vi "rotate_nicks_bot.vi"(8 "degrees to  rotate":dbl, 9 "right(T)/left(F)":bool, 10 "power":u16=75, 11 "NXT 2":T1={"Hardware"="NXT", "Flattened String"=""}) -> (3 "NXT":T1={"Hardware"="NXT", "Flattened String"=""})   [LabVIEW 2012]
uses:
  <vilib>/NXT/Subs/LVHSConnector.ctl
  <vilib>/NXT/Subs/MotorOutput.ctl
  <vilib>/NXT/Dual Mode Library/Motors/MotorBrake.vi
  <vilib>/NXT/Dual Mode Library/Display/drawText.vi
  <vilib>/NXT/Dual Mode Library/Waits/Wait_Num.vi
  <vilib>/NXT/Dual Mode Library/Motors/MotorOn.vi
  <vilib>/NXT/Dual Mode Library/Motors/MotorReverse.vi
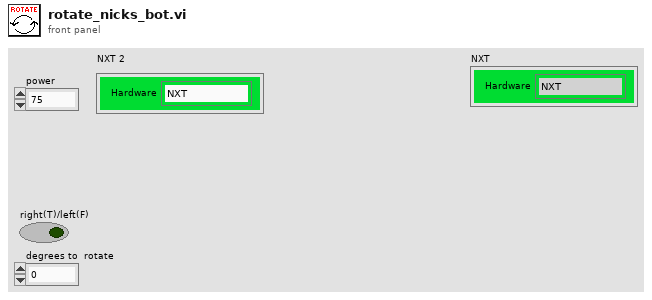
[diagram p1: front panel]
types:
  T1 = typedef "LVHSConnector.ctl" = cluster{"Hardware":string, "Flattened String":string}
  T2 = typedef "MotorOutput.ctl" = u8
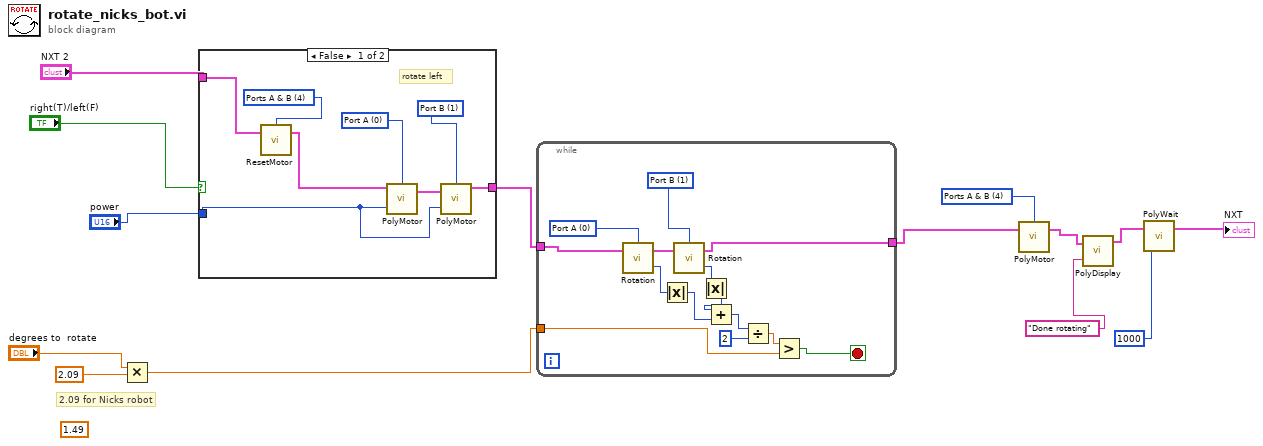
[diagram p0: block diagram]
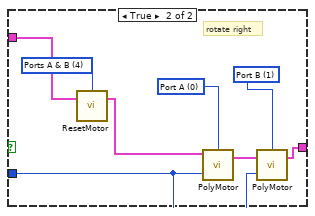
[diagram p2: hidden frame]
diagram:
  (unwired) 1.49 ("Max Value")
  w1 = T2 4 items=["Port A"=0, "Port B"=1, "Port C"=2, "Ports A & B"=4, "Ports A & C"=5, "Ports B & C"=6, "All Ports"=3] ("Port (All Ports)")
  # "2.09 for Nicks robot"
  n1 = Multiply(x="degrees to  rotate", y=2.09 ("Max Value")) -> (x*y=w10:dbl)
  n2 = case shown="False" "right(T)/left(F)" {
    tunnel: "power" -> [w15 w23]
    tunnel: "NXT 2" -> [w19 w25]
    tunnel: [w17 w24] -> w8
    frame False {
      w16 = T2 4 items=["Port A"=0, "Port B"=1, "Port C"=2, "Ports A & B"=4, "Ports A & C"=5, "Ports B & C"=6, "All Ports"=3] ("Port (All Ports)")
      w22 = T2 1 items=["Port A"=0, "Port B"=1, "Port C"=2, "Ports A & B"=4, "Ports A & C"=5, "Ports B & C"=6, "as"=3] ("Output Port (All Ports)")
      w20 = T2 0 items=["Port A"=0, "Port B"=1, "Port C"=2, "Ports A & B"=4, "Ports A & C"=5, "Ports B & C"=6, "as"=3] ("Output Port (All Ports)")
      # "rotate left"
      n3 = call <vilib>:"ResetMotor.vi"("NXT"=w19, "Port (All Ports)"=w16) -> ("NXT"=w18:T1)  [unwired: 2 in]
      n4 = call-poly <vilib>:"PolyMotor.vi"("Power (75)"=w15, "NXT"=w18, "Output Port (All Ports)"=w20) -> ("NXT"=w21:T1)  [unwired: 1 in]
      n5 = call-poly <vilib>:"PolyMotor.vi"("Power (75)"=w15, "NXT"=w21, "Output Port (All Ports)"=w22) -> ("NXT"=w17:T1)  [unwired: 1 in]
    }
    frame True {
      w26 = T2 4 items=["Port A"=0, "Port B"=1, "Port C"=2, "Ports A & B"=4, "Ports A & C"=5, "Ports B & C"=6, "All Ports"=3] ("Port (All Ports)")
      w30 = T2 1 items=["Port A"=0, "Port B"=1, "Port C"=2, "Ports A & B"=4, "Ports A & C"=5, "Ports B & C"=6, "as"=3] ("Output Port (All Ports)")
      w28 = T2 0 items=["Port A"=0, "Port B"=1, "Port C"=2, "Ports A & B"=4, "Ports A & C"=5, "Ports B & C"=6, "as"=3] ("Output Port (All Ports)")
      # "rotate right"
      n6 = call <vilib>:"ResetMotor.vi"("NXT"=w25, "Port (All Ports)"=w26) -> ("NXT"=w27:T1)  [unwired: 2 in]
      n7 = call-poly <vilib>:"PolyMotor.vi"("Power (75)"=w23, "NXT"=w27, "Output Port (All Ports)"=w28) -> ("NXT"=w29:T1)  [unwired: 1 in]
      n8 = call-poly <vilib>:"PolyMotor.vi"("Power (75)"=w23, "NXT"=w29, "Output Port (All Ports)"=w30) -> ("NXT"=w24:T1)  [unwired: 1 in]
    }
  }
  n9 = while {
    tunnel: w8 -> [w44]
    tunnel: w10 -> [w33]
    tunnel: [w40] -> w3
    stop <- w31 stop-if-true
    w41 = T2 1 items=["Port A"=0, "Port B"=1, "Port C"=2, "Ports A & B"=4, "Ports A & C"=5, "Ports B & C"=6, "as"=3] ("Output Port (All Ports)")
    w42 = T2 0 items=["Port A"=0, "Port B"=1, "Port C"=2, "Ports A & B"=4, "Ports A & C"=5, "Ports B & C"=6, "as"=3] ("Output Port (All Ports)")
    n10 = call <vilib>:"Rotation.vi"("NXT"=w44, "Port (Port A)"=w42) -> ("Angle of Rotation"=w39:i32, "NXT"=w43:T1)  [unwired: 1 in]
    n11 = Absolute Value(x=w39) -> (abs(x)=w37:i32)
    n12 = call <vilib>:"Rotation.vi"("NXT"=w43, "Port (Port A)"=w41) -> ("Angle of Rotation"=w38:i32, "NXT"=w40:T1)  [unwired: 1 in]
    n13 = Absolute Value(x=w38) -> (abs(x)=w36:i32)
    n14 = Add(x=w36, y=w37) -> (x+y=w35:i32)
    n15 = Divide(x=w35, y=2) -> (x/y=w32:dbl)
    n16 = Greater?(x=w32, y=w33) -> (0:w31:bool)
  }
  n17 = call-poly <vilib>:"PolyMotor.vi"("NXT"=w3, "Port (All Ports)"=w1) -> ("NXT"=w2:T1)  [unwired: 2 in]
  n18 = call-poly <vilib>:"PolyDisplay.vi"("Text"="Done rotating", "NXT"=w2) -> ("NXT"=w6:T1)  [unwired: 2 in]
  n19 = call-poly <vilib>:"PolyWait.vi"("Time (1 sec)"=u16 1000 ("Max Value"), "NXT"=w6) -> ("NXT"=→"NXT":T1)  [unwired: 2 in]
